vi "update.name.vi"(8 "error in (no error)":errorcluster, 10 "Title":string, 11 "Run in":refnum<class "Run.lvclass">) -> (0 "error out":errorcluster, 3 "Run out":refnum<class "Run.lvclass">)   [LabVIEW 2020, in "Run.lvclass"]
uses:
  Run.lvclass
  Run.lvclass/Run.ctl
  Nominal Client/Nominal Client.lvclass/Nominal Client.ctl
  Nominal Client/error.vi
  Nominal Client/trace.payload_sent.vi
  Nominal Client/trace.payload_received.vi
  Nominal Client/create.authorization_header.vi
  Nominal Client/error.vi/859f8e04-e495-489b-b5b4-7ac163f56130.vi
  Nominal Client/trace.calling_method.vi
  <vilib>/JDP Science/JDP Science Common Utilities/Trim Whitespace__JDP.vi
  <vilib>/AdvancedString/1D String Array to Delimited String.vi
  Nominal Client/api_token.get.vi
  <vilib>/Utility/libraryn.llb/Get File Extension.vi
  Nominal Client/log_file.write.vi
  <vilib>/JDP Science/JSONtext/Get all Object Items.vi
  <vilib>/Utility/error.llb/Error Cluster From Error Code.vi
  <vilib>/JDP Science/JSONtext/JSON text to Variant.vi
  <vilib>/JDP Science/JSONtext/LVClass Serializer/JSONtext LVClass Serializer.lvclass
  <vilib>/addons/_JKI.lib/REST Client/classes/Response Headers/Response Headers.lvclass
  <vilib>/addons/_JKI.lib/REST Client/classes/REST Client/REST Client.lvclass
  Nominal Client/Nominal Client.lvclass
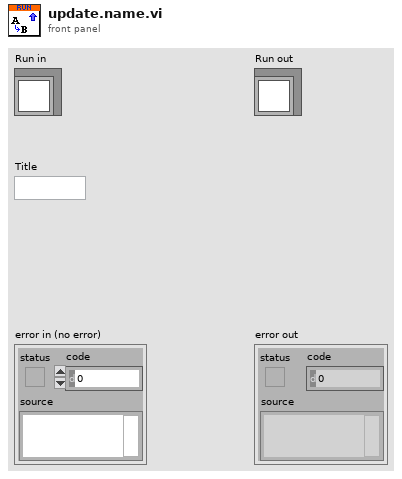
[diagram p1: front panel]
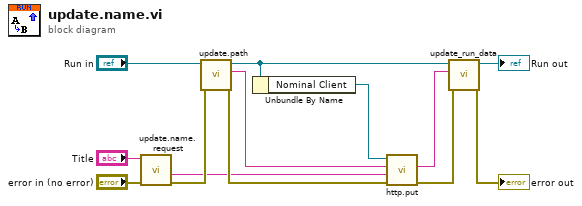
[diagram p0: block diagram]
diagram:
  n1 = call "update.name.request.vi"("error in"="error in (no error)", "Title"="Title") -> ("error out"=w4:errorcluster, "Request"=w2:string)  [unwired: 8 in]
  n2 = call "update.path.vi"("error in"=w4, "Run"="Run in") -> ("error out"=w3:errorcluster, "path"=w10:string, "Run Out"=w9:refnum<class "Run.lvclass">)  [unwired: 7 in]
  n3 = Unbundle By Name(w9) -> ("Nominal Client"=w11:refnum<class "Nominal Client.lvclass">)
  n4 = call "http.put.vi"("error in"=w3, "Body"=w2, "Path"=w10, "Nominal Client in"=w11) -> ("error out"=w8:errorcluster, "Response"=w7:string)  [unwired: 4 in, 2 out]
  n5 = call "update_run_data.vi"("error in"=w8, "Run JSON"=w7, "Run in"=w9) -> ("error out"=→"error out":errorcluster, "Run out"=→"Run out":refnum<class "Run.lvclass">)  [unwired: 7 in]
